vi "RSNRPZ Set Scope Auto Type.vi"(8 "error in (no error)":errorcluster, 9 "Method (Resolution)":i32(ring) items=["Resolution", "Noise Ratio"], 10 "Channel (1)":i32=1, 11 "VISA session":refnum<visa-resource-name> caption="VISA resource name") -> (0 "error out":errorcluster, 3 "dup VISA session":refnum<visa-resource-name> caption="VISA resource name")   [LabVIEW 2010]
doc: "This VI selects a method by which the automatic filter length switchover can operate.\n\nRemote-control command(s):\nSENS:TRAC:AVER:COUN:AUTO:TYPE RES | NSR"
uses:
  rsnrpz_32.dll
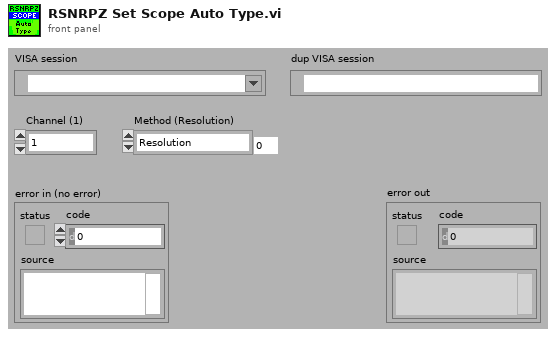
[diagram p1: front panel]
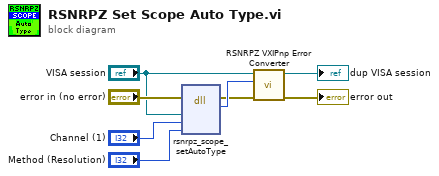
[diagram p0: block diagram]
diagram:
  n1 = dll-call lib="rsnrpz_32.dll" fn="rsnrpz_scope_setAutoType"(error in="error in (no error)", "Instrument Handle"="VISA session", "Channel"="Channel (1)", "Method"="Method (Resolution)") -> (error out=w5:errorcluster, "Status"=w8:i32)  [unwired: 5 in, 1 out]
  n2 = call <instrlib>:"RSNRPZ VXIPnp Error Converter.vi"("error in"=w5, "VXIPnp error code"=w8, "VISA session"="VISA session") -> ("error out"=→"error out":errorcluster, "dup VISA session"=→"dup VISA session":refnum<visa-resource-name>)  [unwired: 7 in]
